vi "ForLoop_Shift_Register.vi"() -> ()   [LabVIEW 2018]
panel:
  out "숫자형 3":i32
  out "숫자형 2":i32
  out "n-3":i32
  out "n-2":i32
  out "n-1":i32
  out "숫자형":i32
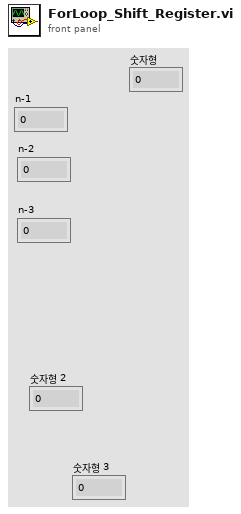
[diagram p1: front panel]
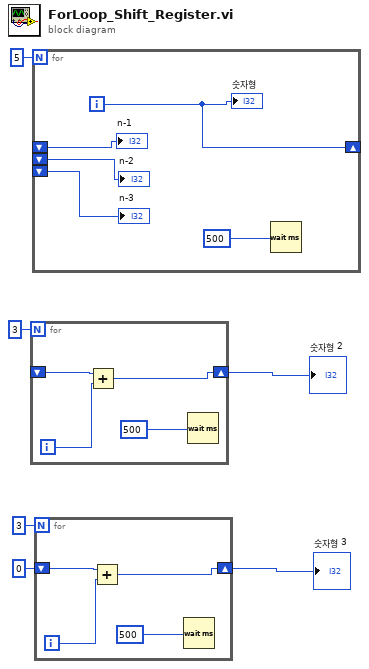
[diagram p0: block diagram]
diagram:
  n1 = for {
    N: 3 -> [_]
    shift-right: [w8] -> w4
    shift-left: _ -> [w9]
    i -> [w10]
    n2 = Add(x=w9, y=w10) -> (x+y=w8:i32)
    n3 = Wait (ms)(milliseconds to wait=500) -> ()  [unwired: 1 out]
  }
  "숫자형 2" <- w4
  n4 = for "For 루프" {
    N: 5 -> [_]
    shift-right: [w14] -> _
    shift-left: _ -> [w15]
    shift-left: _ -> [w13]
    shift-left: _ -> [w12]
    i -> [w14]
    n5 = Wait (ms)(milliseconds to wait=500) -> ()  [unwired: 1 out]
    "숫자형" <- w14
    "n-1" <- w15
    "n-2" <- w13
    "n-3" <- w12
  }
  n6 = for {
    N: 3 -> [_]
    shift-right: [w17] -> w2
    shift-left: 0 -> [w18]
    i -> [w19]
    n7 = Add(x=w18, y=w19) -> (x+y=w17:i32)
    n8 = Wait (ms)(milliseconds to wait=500) -> ()  [unwired: 1 out]
  }
  "숫자형 3" <- w2
